vi "Configure Modulation Low Level (FM State).vi"(8 "error in":errorcluster, 10 "Enable Frequency Modulation (F: Disable)":bool, 11 "VISA resource name":refnum<visa-resource-name>) -> (0 "error out":errorcluster, 3 "VISA resource name out":refnum<visa-resource-name>)   [LabVIEW 2017, in "Keithley 3390.lvlib"]
doc: "Enables or disables the FM modulation technique.\n\n<b>Notes:</b>\nOnly one form of modulation may be active at a time. If one form of modulation is enabled whilst another form is already active, the currently active form will be disable and the newly enabled form will become the active form."
uses:
  Keithley 3390.lvlib
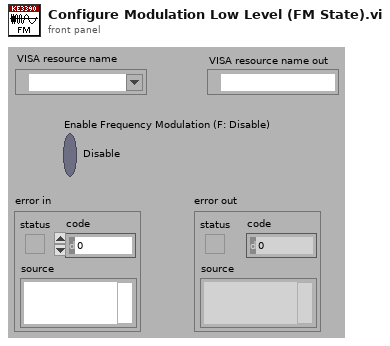
[diagram p1: front panel]
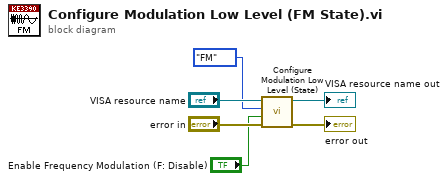
[diagram p0: block diagram]
diagram:
  n1 = call "Configure Modulation Low Level (State).vi"("error in (no error)"="error in", "Enable (F: Off)"="Enable Frequency Modulation (F: Disable)", "Modulation (AM)"=enum16{"AM", "FM", "PM", "FSK", "PWM"}."FM" ("Modulation (0:AM)"), "VISA resource name"="VISA resource name") -> ("error out"=→"error out":errorcluster, "VISA resource name out"=→"VISA resource name out":refnum<visa-resource-name>)  [unwired: 6 in]
